vi "mono_camera_single.vi"(4 "error in":errorcluster, 5 "connection ID":refnum<k5>, 6 "stream dimensions":cluster{"x dimension":dbl, "y dimension":dbl}) -> (0 "error out":errorcluster, 1 "tcp_out":refnum<k5>, 2 "camera_out":picture)   [LabVIEW 2018]
uses:
  monoDrive.lvlib
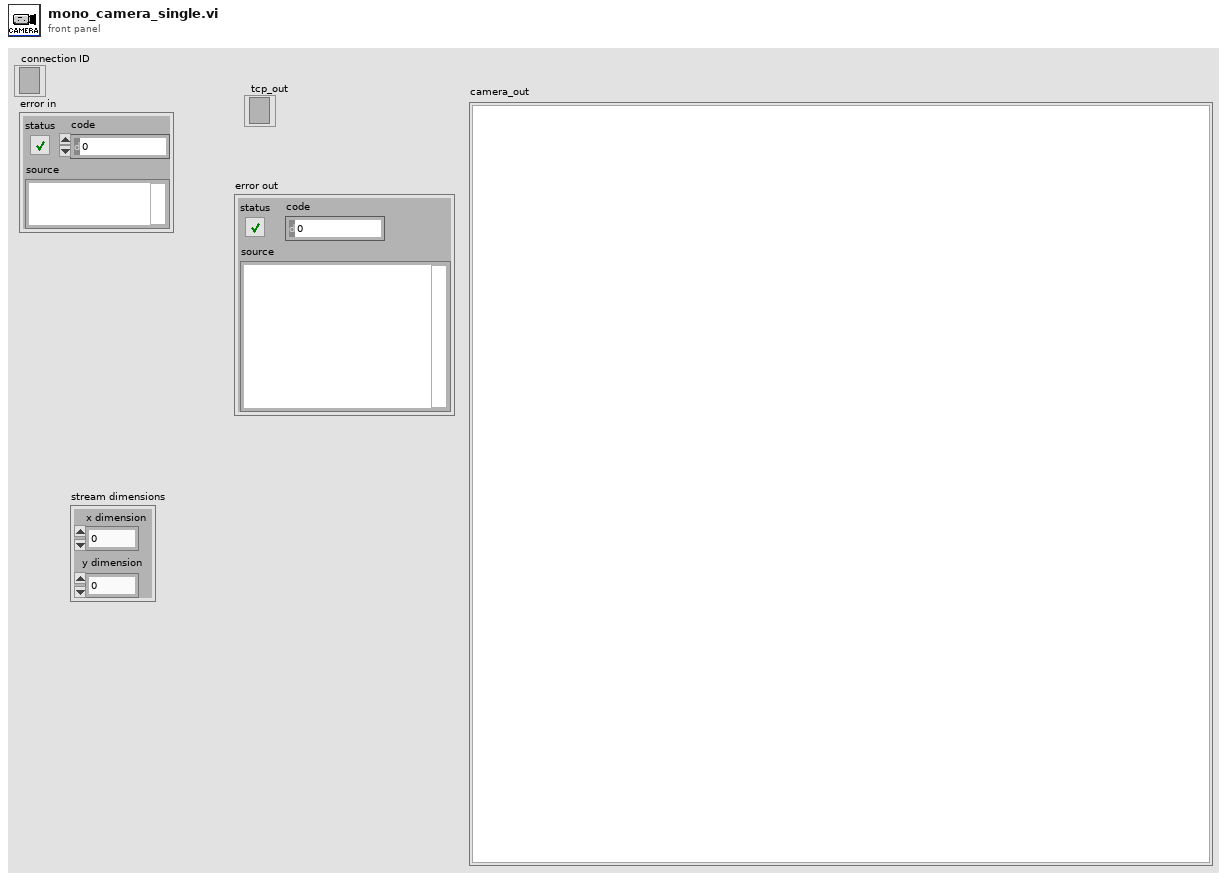
[diagram p1: front panel]
types:
  T1 = cluster{cluster{"length":u32, "time_stamp":u32, "game_time":sgl}, "data out":string}
  T2 = typedef "imagedata.ctl" = cluster{"image type":i32, "image depth":i32, "image":u8[], "mask":u8[], "colors":u32[], "Rectangle":cluster{"left":i16, "top":i16, "right":i16, "bottom":i16}}
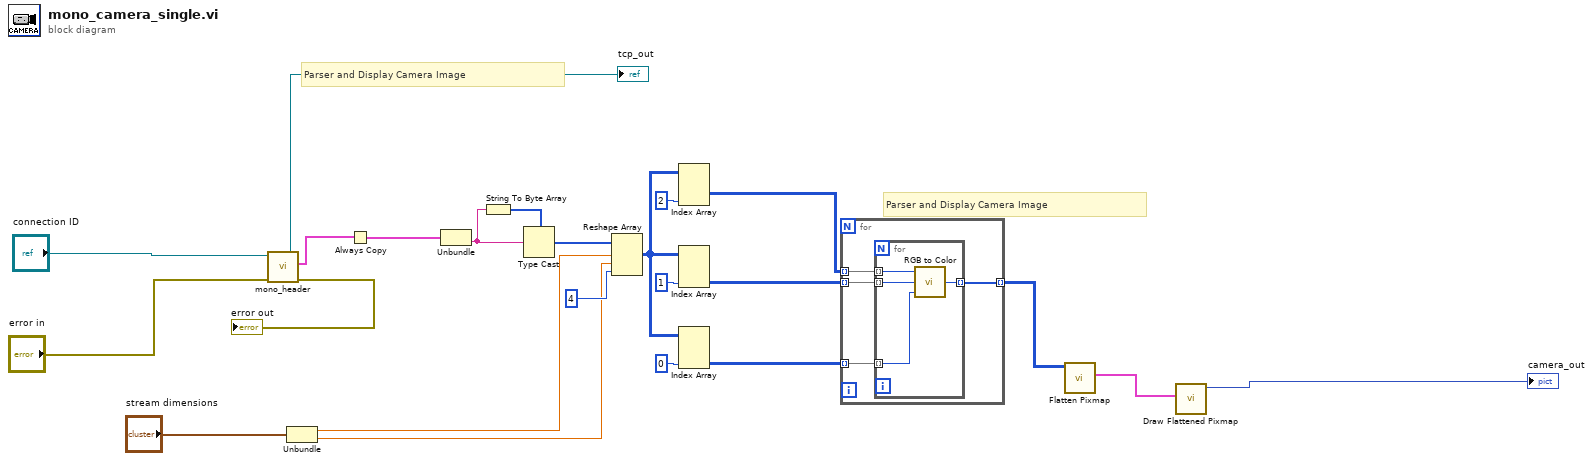
[diagram p0: block diagram]
diagram:
  # "Parser and Display Camera Image"
  # "Parser and Display Camera Image"
  n1 = call "mono_header.vi"("error in"="error in", "connection ID"="connection ID") -> ("error out"=→"error out":errorcluster, "sensor_sample"=w5:T1, "connection ID out"=→"tcp_out":refnum<k5>)  [unwired: 7 in]
  n2 = Unbundle("stream dimensions") -> ("x dimension"=w2:dbl, "y dimension"=w1:dbl)
  n3 = Always Copy(1:w5) -> (0:w6:T1)
  n4 = Unbundle(w6) -> ("data out"=w20:string)  [unwired: 1 out]
  n5 = String To Byte Array(string=w20) -> (unsigned byte array=w21:u8[])
  n6 = Type Cast(type=w21, x=w20) -> (*(type *) &x=w4:u8[])
  n7 = Reshape Array(w4, w2, w1, 4 ("dimension size")) -> (w9:u8[][][])
  n8 = Index Array(array=w9, index (dim 2)=2 ("index (col)")) -> (element=w15:u8[][])  [unwired: 2 in]
  n9 = Index Array(array=w9, index (dim 2)=1 ("index (col)")) -> (element=w14:u8[][])  [unwired: 2 in]
  n10 = Index Array(array=w9, index (dim 2)=0 ("disabled index (col)")) -> (element=w13:u8[][])  [unwired: 2 in]
  n11 = for {
    tunnel: w15 -> [w27] mode=indexing
    tunnel: w14 -> [w26] mode=indexing
    tunnel: w13 -> [w25] mode=indexing
    tunnel: [w24] -> w10 mode=indexing
    n12 = for {
      tunnel: w27 -> [w31] mode=indexing
      tunnel: w26 -> [w30] mode=indexing
      tunnel: w25 -> [w29] mode=indexing
      tunnel: [w28] -> w24 mode=indexing
      n13 = call <vilib>:"RGB to Color.vi"("B"=w29, "G"=w30, "R"=w31) -> ("Color"=w28:u32)
    }
  }
  n14 = call <vilib>:"Flatten Pixmap.vi"("24-bit pixmap"=w10) -> ("image data"=w11:T2)  [unwired: 10 in]
  n15 = call <vilib>:"Draw Flattened Pixmap.vi"("image data"=w11) -> ("new picture"=→"camera_out":picture)  [unwired: 8 in]
